vi "参数设置页.vi"() -> ()   [LabVIEW 2016, in "斯坦道CODMn.lvlib"]
uses:
  <vilib>/Utility/config.llb/NI_LVConfig.lvlib
panel:
  in  "采水泵排液时间/s:":i32
  in  "采水泵沉淀时间/s:":i32
  in  "采水泵润洗时间/s:":i32
  in  "采水泵进样时间/s:":i32
  in  "标度泵计量数 2":dbl
  in  "零点泵计量数 2":dbl
  in  "氢氧化钠:":dbl
  in  "屏蔽负值":bool
  in  "常规版/认证版":enum16{"常规版-酸性", "常规版-碱性", "认证版", "浮台版"}(ring)
  out "稀释倍数解释":string
  in  "CODMn零点核查选择":enum16{"零点核查走纯水管", "零点核查走零漂管"}(ring)
  in  "低量程稀释倍数:":dbl=1.0
  in  "高量程稀释倍数:":dbl=2.0
  in  "零点液自动补测":bool
  in  "跨度液自动补测":bool
  in  "标准液自动补测":bool
  in  "零点液偏差":dbl
  in  "跨度液偏差":dbl
  in  "标准液偏差":dbl
  in  "更换泵管":bool
  in  "跨度值":dbl
  in  "加标回收量程：":enum32{"H", "L", "AUTO"}(ring)=enum."AUTO"
  out "CODMn序列号":string
  out "CODMn软件版本：":string
  in  "标样核查量程选择":enum32{"H", "L", "AUTO"}(ring)=enum."AUTO"
  in  "标样浓度":dbl
  in  "零点核查量程选择":enum32{"H", "L", "AUTO"}(ring)=enum."AUTO"
  in  "零点核查浓度":dbl
  in  "跨度量程选择":enum32{"H", "L", "AUTO"}(ring)=enum."AUTO"
  in  "跨度液浓度":dbl
  in  "水样：":dbl
  in  "蒸馏水：":dbl
  in  "标液：":dbl
  in  "零点核查样：":dbl
  in  "加标回收样：":dbl
  in  "草酸钠":dbl
  in  "高锰酸钾":dbl
  in  "硫酸":dbl
  out "量程解释说明":string
  in  "高切低阈值:":dbl
  in  "低切高阈值:":dbl
  in  "水样量程选择:":enum16{"L", "H", "自动切换测一次", "自动切换测两次"}(ring)
  in  "标准液浓度":dbl
  in  "温度":dbl
  in  "恒温时间":dbl
  in  "当前量程：":enum16{"L", "H"}(ring)
  # "基本参数设置"
  # "泵计量参数设置"
  # "高锰酸钾："
  # "加热恒温温度(℃):"
  # "草酸钠："
  # "恒温时间(分钟):"
  # "硫酸："
  # "标准液浓度(mg/L):"
  # "跨度核查浓度："
  # "零点液偏差±:"
  # "标准液偏差%:"
  # "跨度核查量程："
  # "跨度液偏差%:"
  # "零点核查浓度："
  # "标样浓度："
  # "零点核查量程："
  # "标样核查量程："
  # "跨度值:"
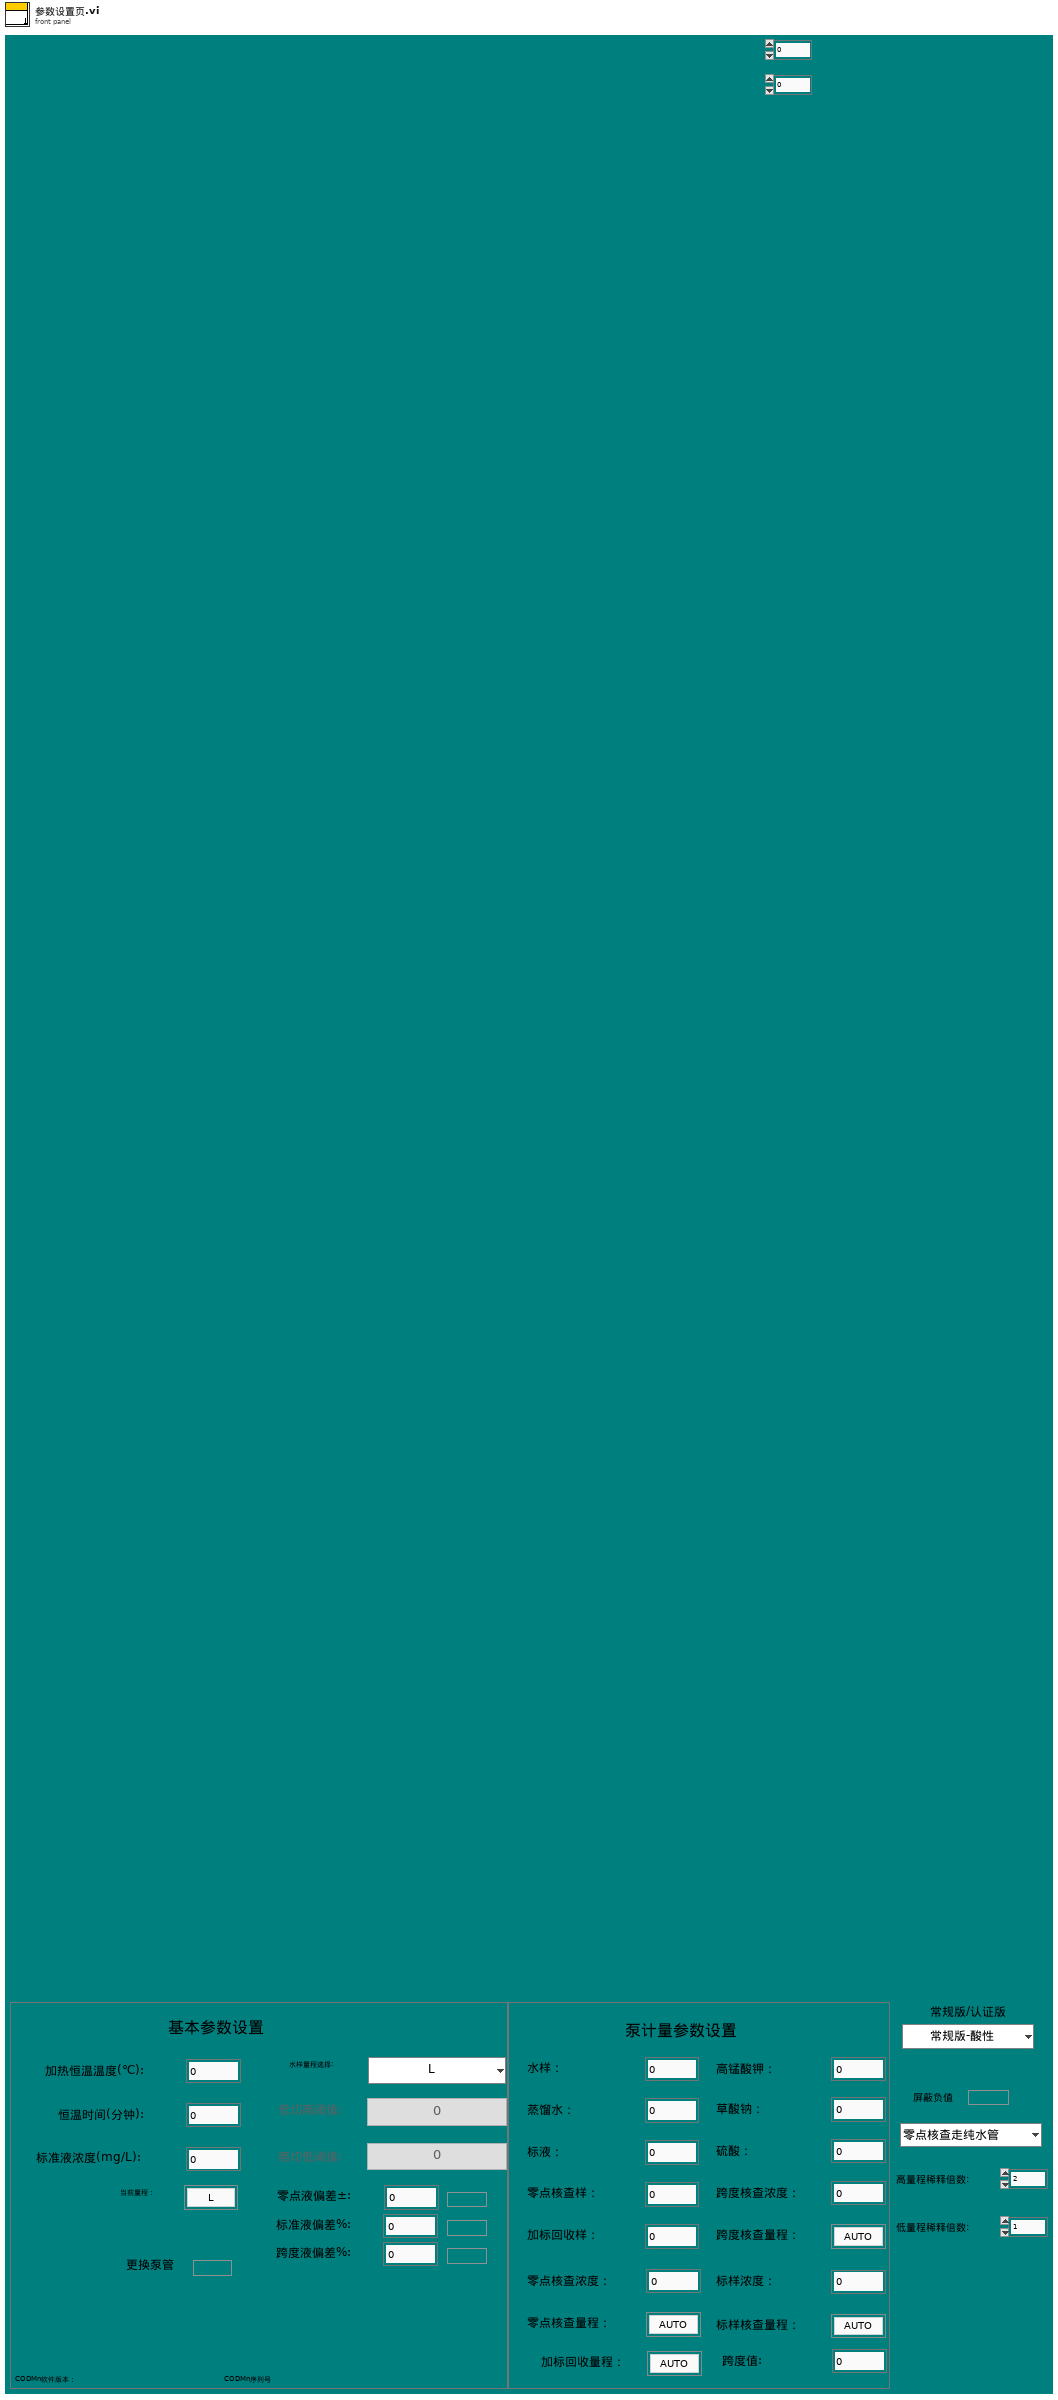
[diagram p1: front panel]
types:
  T1 = typedef "NI_LVConfig.lvlib/Config Data RefNum.ctl" = refnum<k1>
  T2 = cluster{"时间":timestamp, "水样计量数":u16, "蒸馏水计量数":u16, "标液计量数":u16, "零点核查计量数":u16, "加标回收计量数":u16, "硫酸计量数":u16, "高锰酸钾计量数":u16, "草酸钠计量数":u16, "更换泵管":string}
  T3 = cluster{"测量量程":dbl, "测量精度":dbl, "测量间隔":dbl, "消解温度":dbl, "消解时长":dbl, "空白校准时间":timestamp, "曲线截距":dbl, "曲线斜率":dbl, "测量检出限":dbl, "测量信号值":dbl, "线性相关系数":dbl, "二次多项式系数":dbl, "标样校准时间":timestamp, "稀释倍数":dbl, "三项式系数":dbl, "空白标定系数":dbl, "量程系数":dbl, "F0/ORPA":dbl, "F1/ORPB":dbl, "F2/ORPK":dbl, "F3":dbl, "F4":dbl, "F5":dbl, "F6":dbl, "F7":dbl, "X0/滴定数":dbl, "量程":dbl}
  T4 = enum8{"Enabled", "Disabled", "Disabled and Grayed Out"}
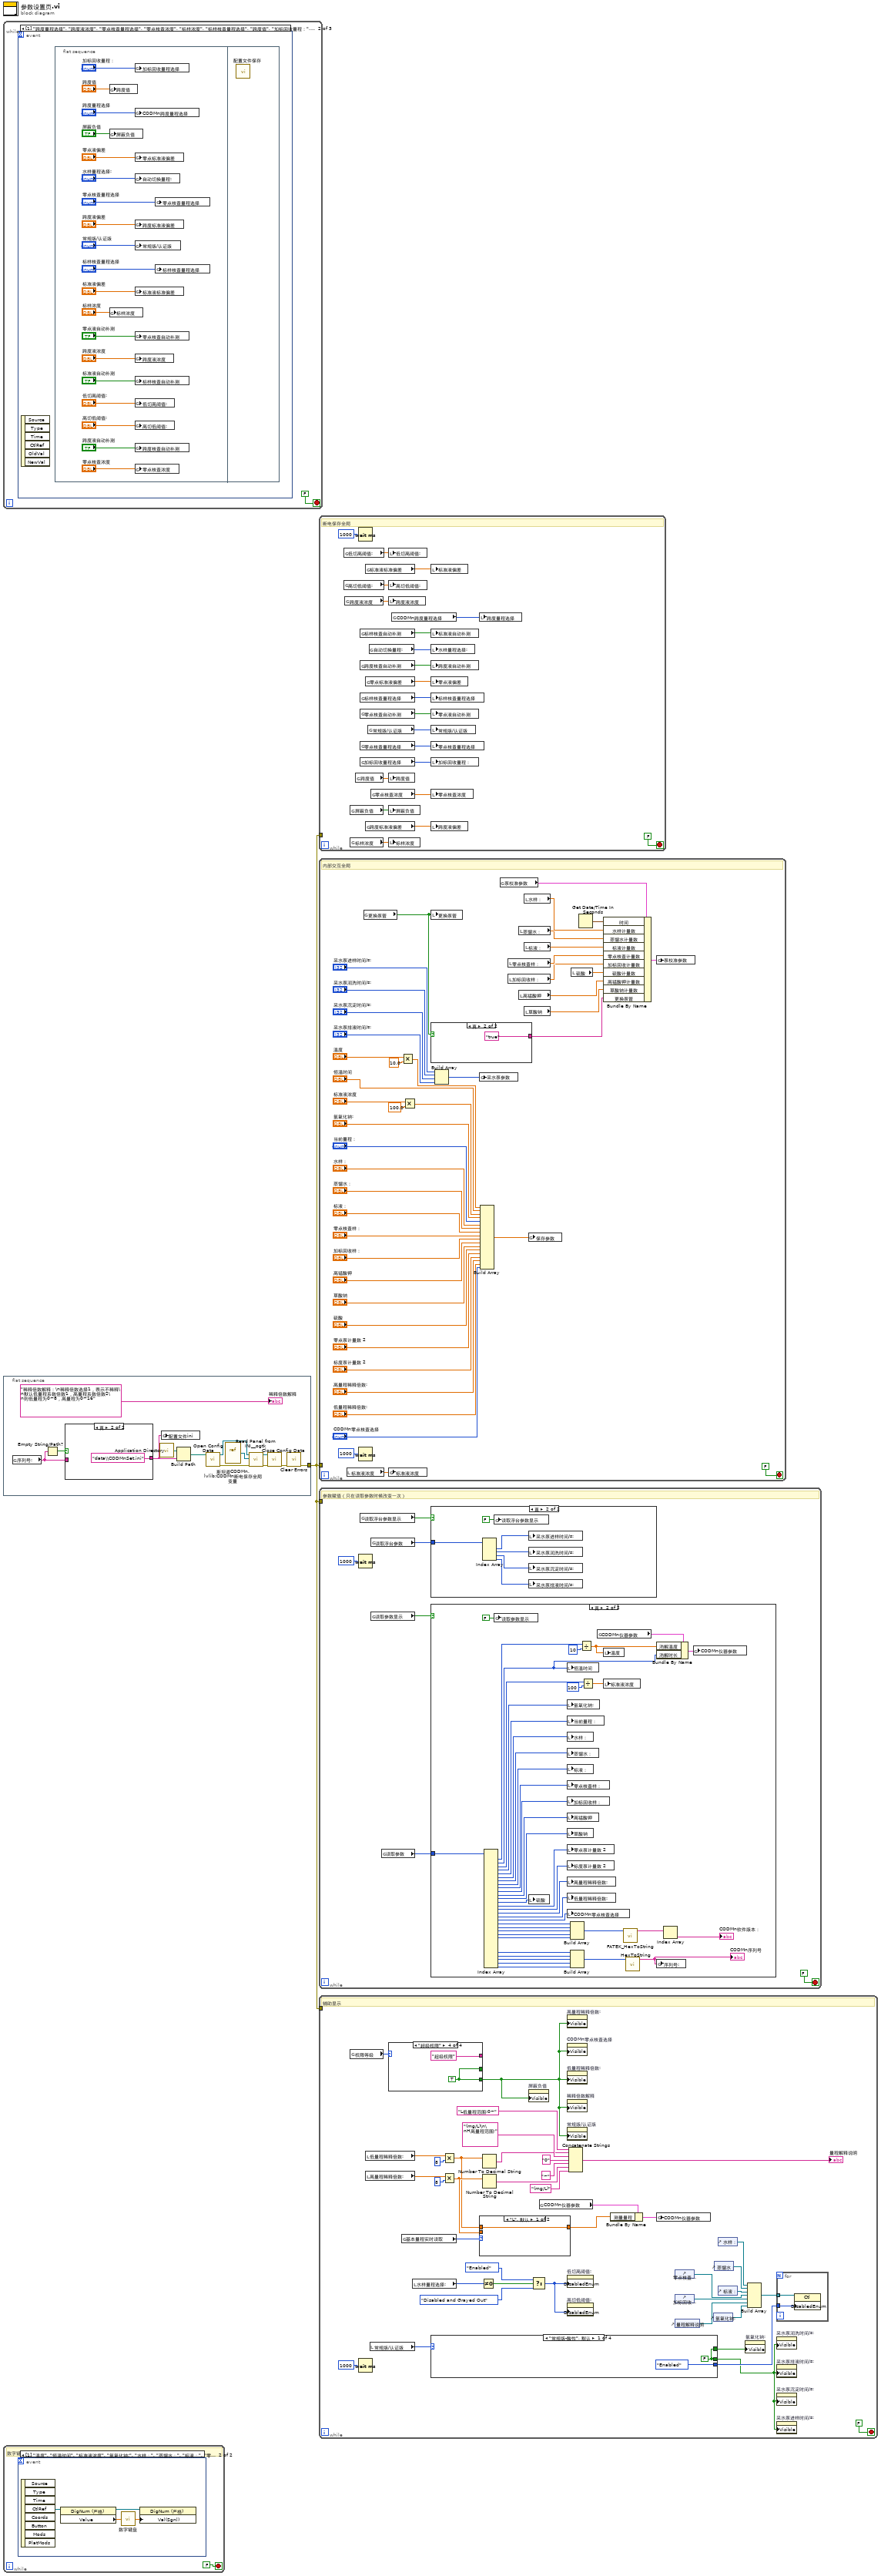
[diagram p0: block diagram]
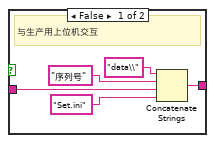
[diagram p2: hidden frame]
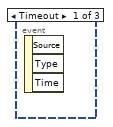
[diagram p3: hidden frame]
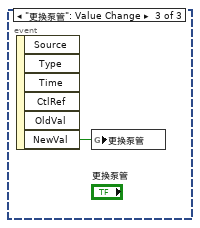
[diagram p4: hidden frame]
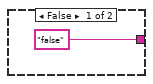
[diagram p7: hidden frame]
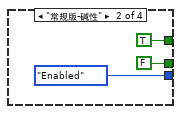
[diagram p8: hidden frame]
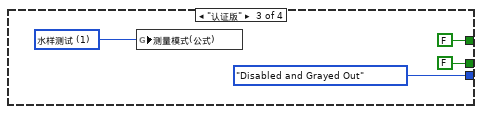
[diagram p9: hidden frame]
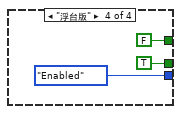
[diagram p10: hidden frame]
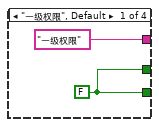
[diagram p11: hidden frame]
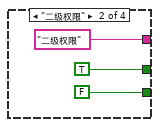
[diagram p12: hidden frame]
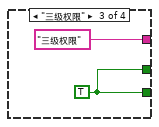
[diagram p13: hidden frame]
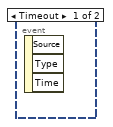
[diagram p15: hidden frame]
diagram:
  n1 = while {
    stop <- FALSE stop-if-true
    n2 = event shown="[1] \"跨度量程选择\", \"跨度液浓度\", \"零点核查量程选择\", \"零点核查浓度\", \"标样浓度\", \"标样核查量程选择\", \"跨度值\", \"加标回收量程：\", \"标准液偏差\", \"跨度液偏差\", \"零点液偏差\", \"标准液自动补测\", \"跨度液自动补测\", \"零点液自动补测\", \"常规版/认证版\", \"屏蔽负值\", \"水样量程选择:\", \"低切高阈值:\", \"高切低阈值:\": 值改变" {
      selector: _ -> [_ _ _]
      dyn-events: _ -> [_ _ _]
      timeout: _ -> [_ _ _]
      event Timeout {
        n3 = event-data() -> ()  [unwired: 1 in, 3 out]
      }
      event "跨度量程选择", "跨度液浓度", "零点核查量程选择", "零点核查浓度", "标样浓度", "标样核查量程选择", "跨度值", "加标回收量程：", "标准液偏差", "跨度液偏差", "零点液偏差", "标准液自动补测", "跨度液自动补测", "零点液自动补测", "常规版/认证版", "屏蔽负值", "水样量程选择:", "低切高阈值:", "高切低阈值:": Value Change {
        n4 = event-data() -> ()  [unwired: 1 in, 6 out]
        n5 = flat-sequence {
          frame #0 {
            n6 = global write "CODMn断电保存全局变量.vi" "跨度值"("跨度值") -> ()
            n7 = global write "CODMn断电保存全局变量.vi" "屏蔽负值"("屏蔽负值") -> ()
            n8 = global write "CODMn断电保存全局变量.vi" "标样浓度"("标样浓度") -> ()
            n9 = global write "CODMn断电保存全局变量.vi" "加标回收量程选择"("加标回收量程：") -> ()
            n10 = global write "CODMn断电保存全局变量.vi" "CODMn跨度量程选择"("跨度量程选择") -> ()
            n11 = global write "CODMn断电保存全局变量.vi" "零点标准液偏差"("零点液偏差") -> ()
            n12 = global write "CODMn断电保存全局变量.vi" "自动切换量程:"("水样量程选择:") -> ()
            n13 = global write "CODMn断电保存全局变量.vi" "跨度标准液偏差"("跨度液偏差") -> ()
            n14 = global write "CODMn断电保存全局变量.vi" "常规版/认证版"("常规版/认证版") -> ()
            n15 = global write "CODMn断电保存全局变量.vi" "标准液标准偏差"("标准液偏差") -> ()
            n16 = global write "CODMn断电保存全局变量.vi" "零点核查自动补测"("零点液自动补测") -> ()
            n17 = global write "CODMn断电保存全局变量.vi" "跨度液浓度"("跨度液浓度") -> ()
            n18 = global write "CODMn断电保存全局变量.vi" "标样核查自动补测"("标准液自动补测") -> ()
            n19 = global write "CODMn断电保存全局变量.vi" "低切高阈值:"("低切高阈值:") -> ()
            n20 = global write "CODMn断电保存全局变量.vi" "高切低阈值:"("高切低阈值:") -> ()
            n21 = global write "CODMn断电保存全局变量.vi" "跨度核查自动补测"("跨度液自动补测") -> ()
            n22 = global write "CODMn断电保存全局变量.vi" "零点核查浓度"("零点核查浓度") -> ()
            n23 = global write "CODMn断电保存全局变量.vi" "零点核查量程选择"("零点核查量程选择") -> ()
            n24 = global write "CODMn断电保存全局变量.vi" "标样核查量程选择"("标样核查量程选择") -> ()
          }
          frame #1 {
            n25 = call "配置文件保存.vi"() -> ()  [unwired: 12 in]
          }
        }
      }
      event "更换泵管": Value Change {
        n26 = event-data() -> ("NewVal"=w22:bool)  [unwired: 1 in, 5 out]
        n27 = global write "COD内部交互全局.vi" "更换泵管"(w22) -> ()
      }
    }
  }
  n28 = flat-sequence {
    tunnel: [w24] -> w1
    frame #0 {
      n29 = global read "COD内部交互全局.vi" "序列号:"() -> (w34:string)
      n30 = Empty String/Path?(string/path=w34) -> (empty?=w25:bool)
      n31 = case shown="真" w25 {
        tunnel: w34 -> [w37 _]
        tunnel: [w36 "data\\CODMnSet.ini" ("名称或相对路径")] -> w28
        frame False {
          # "与生产用上位机交互"
          n32 = Concatenate Strings("data\\" ("字符串"), "序列号" ("字符串"), w37, "Set.ini" ("名称或相对路径")) -> (w36:string)
        }
        frame True {
        }
      }
      n33 = call <vilib>:"Application Directory.vi"() -> ("Application Directory"=w23:path)
      n34 = global write "COD内部交互全局.vi" "配置文件ini"(w28) -> ()
      n35 = Build Path(base path=w23, name or relative path=w28) -> (appended path=w27:path)
      n36 = call <vilib>:"Open Config Data.vi"("configuration file path"=w27) -> ("error out"=w29:errorcluster, "refnum"=w30:T1)  [unwired: 8 in, 1 out]
      n37 = vi-ref "斯坦道CODMn.lvlib:CODMn断电保存全局变量.vi"() -> (w33:refnum<vi>)
      n38 = call <userlib>:"Read Panel from INI__ogtk.vi"("error in (no error)"=w29, "VI ref"=w33, "refnum"=w30) -> ("error out"=w31:errorcluster, "refnum out"=w32:T1)  [unwired: 7 in]
      n39 = call <vilib>:"Close Config Data.vi"("error in (no error)"=w31, "refnum"=w32) -> ("error out"=w26:errorcluster)  [unwired: 8 in, 1 out]
      n40 = call <vilib>:"Clear Errors.vi"("error in (no error)"=w26) -> ("error out"=w24:errorcluster)  [unwired: 5 in, 1 out]
      "稀释倍数解释" <- "稀释倍数解释：\n稀释倍数选择1，表示不稀释\n默认低量程系数倍数1，高量程系数倍数2\n则低量程为0~8，高量程为0~16" ("稀释倍数解释")
    }
  }
  n41 = while {
    stop <- FALSE stop-if-true
    # "数字键盘输入"
    n42 = event shown="[1] \"温度\", \"恒温时间\", \"标准液浓度\", \"氢氧化钠:\", \"水样：\", \"蒸馏水：\", \"标液：\", \"零点核查样：\", \"加标回收样：\", \"草酸钠\", \"高锰酸钾\", \"硫酸\", \"高量程稀释倍数:\", \"低量程稀释倍数:\", \"跨度液浓度\", \"零点核查浓度\", \"标样浓度\", \"标准液偏差\", \"跨度液偏差\", \"零点液偏差\", \"低切高阈值:\", \"高切低阈值:\": 鼠标按下" {
      selector: _ -> [_ _]
      dyn-events: _ -> [_ _]
      timeout: _ -> [_ _]
      event Timeout {
        n43 = event-data() -> ()  [unwired: 1 in, 3 out]
      }
      event "温度", "恒温时间", "标准液浓度", "氢氧化钠:", "水样：", "蒸馏水：", "标液：", "零点核查样：", "加标回收样：", "草酸钠", "高锰酸钾", "硫酸", "高量程稀释倍数:", "低量程稀释倍数:", "跨度液浓度", "零点核查浓度", "标样浓度", "标准液偏差", "跨度液偏差", "零点液偏差", "低切高阈值:", "高切低阈值:": Mouse Down {
        n44 = event-data() -> ("CtlRef"=w46:refnum<vi>)  [unwired: 1 in, 7 out]
        n45 = property class="DigNum (严格)"(reference=w46) -> (reference out=w44:refnum<vi>, "Value"=w45:dbl)  [unwired: 1 in, 1 out]
        n46 = call "数字键盘.vi"("OldNumber"=w45) -> ("NewNumber"=w43:sgl)
        n47 = property class="DigNum (严格)"(reference=w44, "Val(Sgnl)"=w43) -> ()  [unwired: 1 in, 2 out]
      }
    }
  }
  n48 = while {
    tunnel: w1 -> [_]
    stop <- FALSE stop-if-true
    # "断电保存全局"
    n49 = global read "CODMn断电保存全局变量.vi" "低切高阈值:"() -> (w65:dbl)
    n50 = global read "CODMn断电保存全局变量.vi" "高切低阈值:"() -> (w64:dbl)
    n51 = global read "CODMn断电保存全局变量.vi" "跨度液浓度"() -> (w48:dbl)
    n52 = global read "CODMn断电保存全局变量.vi" "屏蔽负值"() -> (w59:bool)
    n53 = global read "CODMn断电保存全局变量.vi" "标样浓度"() -> (w47:dbl)
    n54 = global read "CODMn断电保存全局变量.vi" "跨度值"() -> (w49:dbl)
    n55 = Wait (ms)(milliseconds to wait=u32 1000 ("等待时间（毫秒）")) -> ()  [unwired: 1 out]
    n56 = global read "CODMn断电保存全局变量.vi" "标样核查自动补测"() -> (w57:bool)
    n57 = global read "CODMn断电保存全局变量.vi" "跨度核查自动补测"() -> (w56:bool)
    n58 = global read "CODMn断电保存全局变量.vi" "标样核查量程选择"() -> (w62:enum32{"H", "L", "AUTO"})
    n59 = global read "CODMn断电保存全局变量.vi" "零点核查自动补测"() -> (w58:bool)
    n60 = global read "CODMn断电保存全局变量.vi" "零点核查量程选择"() -> (w52:enum32{"H", "L", "AUTO"})
    n61 = global read "CODMn断电保存全局变量.vi" "加标回收量程选择"() -> (w51:enum32{"H", "L", "AUTO"})
    n62 = global read "CODMn断电保存全局变量.vi" "标准液标准偏差"() -> (w55:dbl)
    n63 = global read "CODMn断电保存全局变量.vi" "零点标准液偏差"() -> (w54:dbl)
    n64 = global read "CODMn断电保存全局变量.vi" "跨度标准液偏差"() -> (w53:dbl)
    n65 = global read "CODMn断电保存全局变量.vi" "常规版/认证版"() -> (w60:enum16{"常规版-酸性", "常规版-碱性", "认证版", "浮台版"})
    n66 = global read "CODMn断电保存全局变量.vi" "自动切换量程:"() -> (w63:enum16{"L", "H", "自动切换测一次", "自动切换测两次"})
    n67 = global read "CODMn断电保存全局变量.vi" "零点核查浓度"() -> (w50:dbl)
    n68 = local write "低切高阈值:"(w65) -> ()
    n69 = local write "高切低阈值:"(w64) -> ()
    n70 = local write "跨度液浓度"(w48) -> ()
    n71 = local write "跨度值"(w49) -> ()
    n72 = local write "屏蔽负值"(w59) -> ()
    n73 = local write "标样浓度"(w47) -> ()
    n74 = global read "CODMn断电保存全局变量.vi" "CODMn跨度量程选择"() -> (w61:enum32{"H", "L", "AUTO"})
    n75 = local write "标准液偏差"(w55) -> ()
    n76 = local write "标准液自动补测"(w57) -> ()
    n77 = local write "水样量程选择:"(w63) -> ()
    n78 = local write "跨度液自动补测"(w56) -> ()
    n79 = local write "零点液偏差"(w54) -> ()
    n80 = local write "标样核查量程选择"(w62) -> ()
    n81 = local write "零点液自动补测"(w58) -> ()
    n82 = local write "常规版/认证版"(w60) -> ()
    n83 = local write "零点核查量程选择"(w52) -> ()
    n84 = local write "加标回收量程："(w51) -> ()
    n85 = local write "零点核查浓度"(w50) -> ()
    n86 = local write "跨度液偏差"(w53) -> ()
    n87 = local write "跨度量程选择"(w61) -> ()
  }
  n88 = while {
    tunnel: w1 -> [_]
    stop <- FALSE stop-if-true
    # "内部交互全局"
    n89 = local read "标准液浓度"() -> (w109:dbl)
    n90 = Wait (ms)(milliseconds to wait=u32 1000 ("等待时间（毫秒）")) -> ()  [unwired: 1 out]
    n91 = global read "COD内部交互全局.vi" "更换泵管"() -> (w68:bool)
    n92 = global write "COD浓度全局变量.vi" "标准液浓度"(w109) -> ()
    n93 = Multiply(x="温度", y=10.0) -> (x*y=w89:dbl)
    n94 = Multiply(x="标准液浓度", y=100.0) -> (x*y=w91:dbl)
    n95 = local write "更换泵管"(w68) -> ()
    n96 = case shown="真" w68 {
      tunnel: ["false" "true"] -> w77
      frame False {
      }
      frame True {
      }
    }
    n97 = Build Array("采水泵进样时间/s:", "采水泵润洗时间/s:", "采水泵沉淀时间/s:", "采水泵排液时间/s:") -> (w85:i32[])
    n98 = global write "COD内部交互全局.vi" "采水泵参数"(w85) -> ()
    n99 = Build Array(w89, "恒温时间", w91, "氢氧化钠:", "当前量程：", "水样：", "蒸馏水：", "标液：", "零点核查样：", "加标回收样：", "高锰酸钾", "草酸钠", "硫酸", "零点泵计量数 2", "标度泵计量数 2", "高量程稀释倍数:", "低量程稀释倍数:", "CODMn零点核查选择") -> (w92:dbl[])
    n100 = global read "COD内部交互全局.vi" "泵校准参数"() -> (w80:T2)
    n101 = local read "零点核查样："() -> (w73:dbl)
    n102 = local read "加标回收样："() -> (w72:dbl)
    n103 = local read "蒸馏水："() -> (w75:dbl)
    n104 = local read "高锰酸钾"() -> (w70:dbl)
    n105 = local read "水样："() -> (w76:dbl)
    n106 = local read "标液："() -> (w74:dbl)
    n107 = local read "草酸钠"() -> (w69:dbl)
    n108 = global write "COD内部交互全局.vi" "保存参数"(w92) -> ()
    n109 = local read "硫酸"() -> (w71:dbl)
    n110 = Get Date/Time In Seconds() -> (seconds since 1Jan1904=w78:timestamp)
    n111 = Bundle By Name(cluster=w80, "时间"=w78, "水样计量数"=w76, "蒸馏水计量数"=w75, "标液计量数"=w74, "零点核查计量数"=w73, "加标回收计量数"=w72, "硫酸计量数"=w71, "高锰酸钾计量数"=w70, "草酸钠计量数"=w69, "更换泵管"=w77) -> (w79:T2)
    n112 = global write "COD内部交互全局.vi" "泵校准参数"(w79) -> ()
  }
  n113 = while {
    tunnel: w1 -> [_]
    stop <- FALSE stop-if-true
    # "参数赋值（只在读取参数时候改变一次）"
    n114 = Wait (ms)(milliseconds to wait=u32 1000 ("等待时间（毫秒）")) -> ()  [unwired: 1 out]
    n115 = global read "COD内部交互全局.vi" "读取浮台参数显示"() -> (w118:bool)
    n116 = global read "COD内部交互全局.vi" "读取浮台参数"() -> (w117:u16[])
    n117 = global read "COD内部交互全局.vi" "读取参数显示"() -> (w115:bool)
    n118 = global read "COD内部交互全局.vi" "读取参数"() -> (w114:u16[])
    n119 = case shown="真" w118 {
      tunnel: w117 -> [_ w165]
      frame False {
      }
      frame True {
        n120 = Index Array(array=w165) -> (element #1=w164:u16, element #2=w163:u16, element #3=w162:u16, element #4=w161:u16)  [unwired: 4 in]
        n121 = global write "COD内部交互全局.vi" "读取浮台参数显示"(FALSE ("读取参数显示")) -> ()
        n122 = local write "采水泵进样时间/s:"(w164) -> ()
        n123 = local write "采水泵润洗时间/s:"(w163) -> ()
        n124 = local write "采水泵沉淀时间/s:"(w162) -> ()
        n125 = local write "采水泵排液时间/s:"(w161) -> ()
      }
    }
    n126 = case shown="真" w115 {
      tunnel: w114 -> [_ w159]
      frame False {
      }
      frame True {
        n127 = Index Array(array=w159) -> (element #1=w157:u16, element #2=w153:u16, element #3=w151:u16, element #4=w149:u16, element #5=w148:u16, element #6=w147:u16, element #7=w146:u16, element #8=w145:u16, element #9=w144:u16, element #10=w143:u16, element #11=w142:u16, element #12=w141:u16, element #13=w140:u16, element #14=w139:u16, element #15=w138:u16, element #16=w137:u16, element #17=w136:u16, element #18=w130:u16, element #19=w129:u16, element #20=w128:u16, element #21=w127:u16, element #22=w126:u16, element #23=w125:u16, element #27=w124:u16, element #28=w123:u16, element #29=w122:u16, element #30=w121:u16, element #31=w120:u16)  [unwired: 31 in, 3 out]
        n128 = global write "COD内部交互全局.vi" "读取参数显示"(FALSE ("读取参数显示")) -> ()
        n129 = local write "硫酸"(w140) -> ()
        n130 = local write "恒温时间"(w153) -> ()
        n131 = local write "氢氧化钠:"(w149) -> ()
        n132 = local write "当前量程："(w148) -> ()
        n133 = local write "水样："(w147) -> ()
        n134 = local write "蒸馏水："(w146) -> ()
        n135 = local write "标液："(w145) -> ()
        n136 = local write "零点核查样："(w144) -> ()
        n137 = local write "加标回收样："(w143) -> ()
        n138 = local write "高锰酸钾"(w142) -> ()
        n139 = local write "草酸钠"(w141) -> ()
        n140 = local write "零点泵计量数 2"(w139) -> ()
        n141 = local write "标度泵计量数 2"(w138) -> ()
        n142 = local write "高量程稀释倍数:"(w137) -> ()
        n143 = local write "低量程稀释倍数:"(w136) -> ()
        n144 = local write "CODMn零点核查选择"(w130) -> ()
        n145 = Build Array(w129, w128, w127, w126, w125) -> (w135:u16[])
        n146 = Build Array(w124, w123, w122, w121, w120) -> (w134:u16[])
        n147 = Divide(x=w157, y=u16 10) -> (x/y=w154:dbl)
        n148 = Divide(x=w151, y=u16 100) -> (x/y=w150:dbl)
        n149 = global read "CODMn断电保存全局变量.vi" "CODMn仪器参数"() -> (w156:T3)
        n150 = local write "温度"(w154) -> ()
        n151 = local write "标准液浓度"(w150) -> ()
        n152 = call "FATEK_HexToString.vi"("数组"=w135) -> ("STRING"=w133:string[])  [unwired: 10 in]
        n153 = call "HexToString.vi"("数组"=w134) -> ("字符串"=w131:string)  [unwired: 10 in]
        "CODMn序列号" <- w131
        n154 = Bundle By Name(cluster=w156, "消解温度"=w154, "消解时长"=w153) -> (w155:T3)
        n155 = global write "COD内部交互全局.vi" "序列号:"(w131) -> ()
        n156 = Index Array(array=w133) -> (element=→"CODMn软件版本：":string)  [unwired: 1 in]
        n157 = global write "CODMn断电保存全局变量.vi" "CODMn仪器参数"(w155) -> ()
      }
    }
  }
  n158 = while {
    tunnel: w1 -> [_]
    stop <- FALSE stop-if-true
    # "辅助显示"
    n159 = global read "CODMN外部API.vi" "权限等级"() -> (w185:enum16{"一级权限", "二级权限", "三级权限", "超级权限"})
    n160 = Wait (ms)(milliseconds to wait=u32 1000 ("等待时间（毫秒）")) -> ()  [unwired: 1 out]
    n161 = local read "低量程稀释倍数:"() -> (w201:dbl)
    n162 = local read "高量程稀释倍数:"() -> (w193:dbl)
    n163 = local read "常规版/认证版"() -> (w175:enum16{"常规版-酸性", "常规版-碱性", "认证版", "浮台版"})
    n164 = case shown="\"超级权限\"" w185 {
      tunnel: [w220 FALSE w225 w227] -> w184
      tunnel: ["一级权限" "二级权限" "三级权限" "超级权限"] -> _
      tunnel: [w220 TRUE w225 w227] -> _
      frame "一级权限", Default {
        w220 = FALSE
      }
      frame "二级权限" {
      }
      frame "三级权限" {
        w225 = TRUE
      }
      frame "超级权限" {
        w227 = TRUE
      }
    }
    n165 = global read "COD内部交互全局.vi" "基本量程实时读取"() -> (w189:enum16{"L", "H", "AUTO"})
    n166 = local read "水样量程选择:"() -> (w168:enum16{"L", "H", "自动切换测一次", "自动切换测两次"})
    n167 = case shown="\"常规版-酸性\", 默认" w175 {
      tunnel: [T4."Enabled" ("禁用") T4."Enabled" ("禁用") T4."Disabled and Grayed Out" ("禁用") T4."Enabled" ("禁用")] -> w174
      tunnel: [w206 TRUE FALSE FALSE] -> w173
      tunnel: [w206 FALSE FALSE TRUE] -> w172
      frame "常规版-酸性", Default {
        w206 = FALSE
      }
      frame "常规版-碱性" {
      }
      frame "认证版" {
        w213 = u16 1 items=["水样测试"=1, "标样核查"=2, "零点核查"=3, "跨度核查"=4, "空白测试"=5, "平行样"=6, "加标回收"=7] ("测量模式(公式)")
        n168 = global write "CODMn断电保存全局变量.vi" "测量模式(公式)"(w213) -> ()
      }
      frame "浮台版" {
      }
    }
    n169 = Multiply(x=w201, y=i8 8) -> (x*y=w187:dbl)
    n170 = Multiply(x=w193, y=i8 8) -> (x*y=w188:dbl)
    n171 = case shown="\"L\", 默认" w189 {
      tunnel: w188 -> [_ w230]
      tunnel: [w229 w230] -> w186
      tunnel: w187 -> [w229 _]
      frame "L", Default {
      }
      frame "H" {
      }
    }
    n172 = Not Equal To 0?(x=w168) -> (x != 0?=w169:bool)
    n173 = Number To Decimal String(number=w187) -> (decimal integer string=w198:string)  [unwired: 1 in]
    n174 = Number To Decimal String(number=w188) -> (decimal integer string=w196:string)  [unwired: 1 in]
    n175 = property on="屏蔽负值" class="Bool (严格)"("Visible"=w184) -> ()  [unwired: 2 in, 2 out]
    n176 = Select(t=T4."Enabled" ("禁用"), s=w169, f=T4."Disabled and Grayed Out" ("禁用")) -> (s? t:f=w167:T4)
    n177 = global read "CODMn断电保存全局变量.vi" "CODMn仪器参数"() -> (w191:T3)
    n178 = property on="高量程稀释倍数:" class="DigNum (严格)"("Visible"=w184) -> ()  [unwired: 2 in, 2 out]
    n179 = property on="CODMn零点核查选择" class="Enum (严格)"("Visible"=w184) -> ()  [unwired: 2 in, 2 out]
    n180 = property on="低量程稀释倍数:" class="DigNum (严格)"("Visible"=w184) -> ()  [unwired: 2 in, 2 out]
    n181 = property on="稀释倍数解释" class="Str"("Visible"=w184) -> ()  [unwired: 2 in, 2 out]
    n182 = property on="常规版/认证版" class="Enum (严格)"("Visible"=w184) -> ()  [unwired: 2 in, 2 out]
    n183 = property on="低切高阈值:" class="DigNum (严格)"("DisabledEnum"=w167) -> ()  [unwired: 2 in, 2 out]
    n184 = property on="高切低阈值:" class="DigNum (严格)"("DisabledEnum"=w167) -> ()  [unwired: 2 in, 2 out]
    n185 = Concatenate Strings("L低量程范围:0~" ("量程解释说明"), w198, "(mg/L)\n\nH高量程范围:" ("量程解释说明"), "0" ("字符串"), "~" ("量程解释说明"), w196, "(mg/L)" ("量程解释说明")) -> (→"量程解释说明":string)
    n186 = Bundle By Name(cluster=w191, "测量量程"=w186) -> (w190:T3)
    n187 = global write "CODMn断电保存全局变量.vi" "CODMn仪器参数"(w190) -> ()
    n188 = control-ref of="零点核查样："() -> (w180:refnum<vi>)
    n189 = control-ref of="加标回收样："() -> (w179:refnum<vi>)
    n190 = control-ref of="量程解释说明"() -> (w178:refnum<vi>)
    n191 = control-ref of="氢氧化钠:"() -> (w177:refnum<vi>)
    n192 = control-ref of="蒸馏水："() -> (w182:refnum<vi>)
    n193 = control-ref of="水样："() -> (w183:refnum<vi>)
    n194 = control-ref of="标液："() -> (w181:refnum<vi>)
    n195 = property on="氢氧化钠:" class="DigNum (严格)"("Visible"=w173) -> ()  [unwired: 2 in, 2 out]
    n196 = Build Array(w183, w182, w181, w180, w179, w178, w177) -> (w176:refnum<vi>[])
    n197 = for {
      tunnel: w176 -> [w219] mode=indexing
      tunnel: w174 -> [w218]
      n198 = property class="Ctl"(reference=w219, "DisabledEnum"=w218) -> ()  [unwired: 1 in, 2 out]
    }
    n199 = property on="采水泵润洗时间/s:" class="DigNum (严格)"("Visible"=w172) -> ()  [unwired: 2 in, 2 out]
    n200 = property on="采水泵排液时间/s:" class="DigNum (严格)"("Visible"=w172) -> ()  [unwired: 2 in, 2 out]
    n201 = property on="采水泵沉淀时间/s:" class="DigNum (严格)"("Visible"=w172) -> ()  [unwired: 2 in, 2 out]
    n202 = property on="采水泵进样时间/s:" class="DigNum (严格)"("Visible"=w172) -> ()  [unwired: 2 in, 2 out]
  }
